vi "Execute.vi"(8 "error in (no error)":errorcluster, 9 "Workspace":T1, 10 "Control In":T2={"I-O.lvclass"=refnum, "Gantry"=refnum, "Dispenser"="COM1"}, 11 "Secure Syringe in":refnum<class "SecureRelease Syringe.lvclass">) -> (0 "error out":errorcluster, 2 "Control Out":T2={"I-O.lvclass"=refnum, "Gantry"=refnum, "Dispenser"="COM1"}, 3 "Secure Syringe out":refnum<class "SecureRelease Syringe.lvclass">)   [LabVIEW 2020, in "SecureRelease Syringe.lvclass"]
uses:
  SecureRelease Syringe.lvclass
  Controller/Controllers.ctl
  Controller/I-O/I-O.lvclass
  C:/Program Files (x86)/Aerotech/A3200/LabVIEW/2010/Bin/Aerotech.A3200.dll
  Program Files (x86)/Aerotech/A3200/LabVIEW/2010/Bin/Aerotech.A3200.dll
  Workspace/Workspace.ctl
  SecureRelease Syringe.lvclass/SecureRelease Syringe.ctl
  Controller/Motion/Motion.lvclass
  Dispense/Dispense.lvclass
  Controller/Motion/A3200/A3200.lvclass
  Controller/Dispenser/Dispenser.lvclass
  Controller/Controller.lvclass
  Workspace/Fixture.lvclass
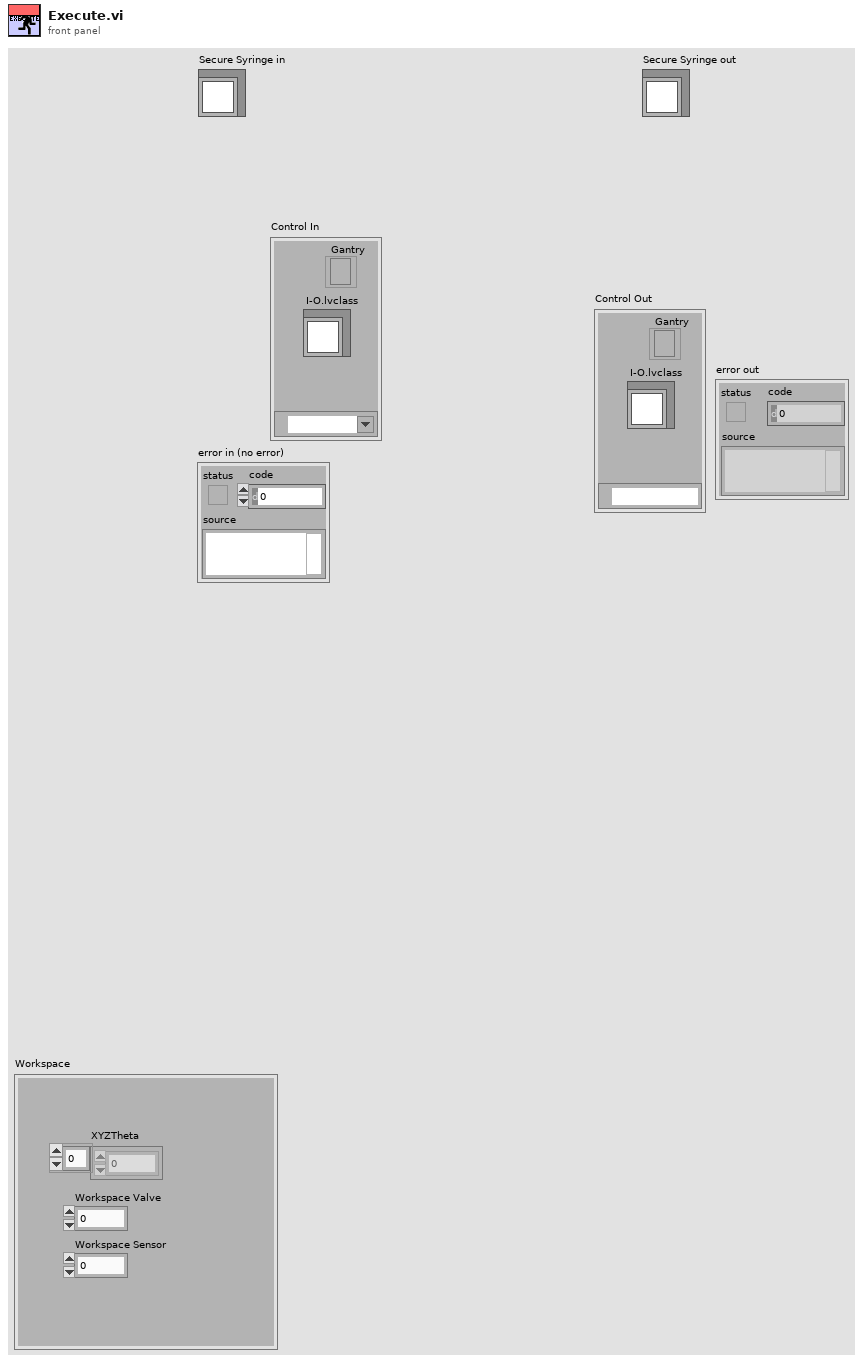
[diagram p1: front panel]
types:
  T1 = typedef "Fixture.lvclass/Workspace.ctl" = cluster{"XYZTheta":dbl[], "Workspace Valve":i32, "Workspace Sensor":i32}
  T2 = typedef "Controller.lvclass/Controllers.ctl" = cluster{"I-O.lvclass":refnum<class "I-O.lvclass">, "Gantry":refnum<k24>, "Dispenser":refnum<visa-resource-name>}
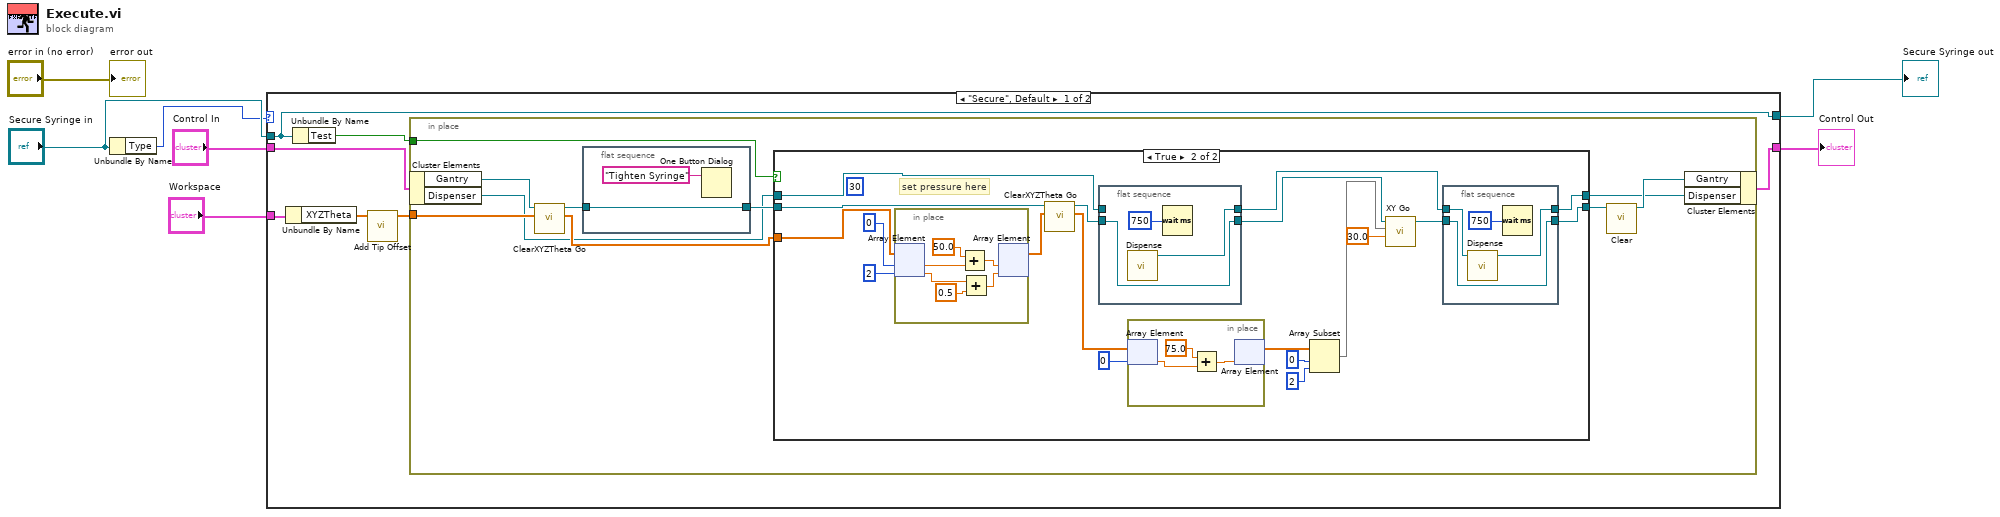
[diagram p0: block diagram]
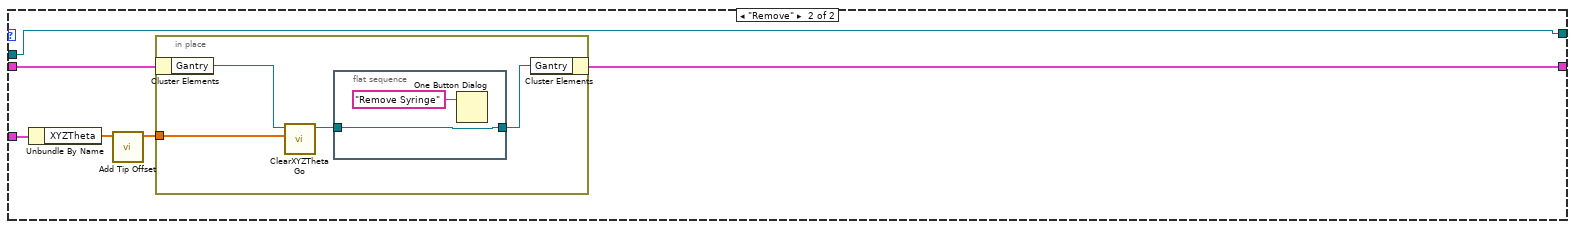
[diagram p3: hidden frame]
diagram:
  n1 = Unbundle By Name("Secure Syringe in") -> ("Type"=w1:enum16{"Secure", "Remove"})
  n2 = case shown="\"Secure\", Default" w1 {
    tunnel: "Workspace" -> [w14 w66]
    tunnel: "Secure Syringe in" -> [w10 w67]
    tunnel: [w10 w67] -> w5
    tunnel: "Control In" -> [w13 w68]
    tunnel: [w12 w69] -> w3
    frame "Secure", Default {
      n3 = Unbundle By Name(w14) -> ("XYZTheta"=w9:dbl[])
      n4 = Unbundle By Name(w10) -> ("Test"=w11:bool)
      n5 = call "Add Tip Offset.vi"("XYZTheta"=w9) -> ("XYZTheta"=w8:dbl[])  [unwired: 10 in]
      n6 = in-place {
        in-place-border: w8 -> [w23]
        in-place-border: w11 -> [w17]
        n7 = in-place-cluster #1(w13) -> ("Gantry"=w24:refnum<k24>, "Dispenser"=w16:refnum<visa-resource-name>)
        n8 = call "ClearXYZTheta Go.vi"("XYZTheta In"=w23, "Gantry In"=w24) -> ("XYZTheta Out"=w18:dbl[], "Gantry Out"=w22:refnum<k24>)  [unwired: 7 in, 1 out]
        n9 = flat-sequence {
          tunnel: [w62] -> w20
          tunnel: w22 -> [w62]
          frame #0 {
            n10 = One Button Dialog(message="Tighten Syringe") -> ()  [unwired: 1 in, 1 out]
          }
        }
        n11 = case shown="True" w17 {
          tunnel: w20 -> [w26 w45]
          tunnel: [w26 w37] -> w19
          tunnel: w18 -> [_ w44]
          tunnel: w16 -> [w25 w27]
          tunnel: [w25 w35] -> w15
          frame False {
          }
          frame True {
            (unwired) i16 30 ("Pressure")
            # "set pressure here"
            n12 = in-place {
              n13 = in-place-array #2(w44, 0, 2) -> (w61:dbl, w59:dbl)
              n14 = Add(x=50.0, y=w61) -> (x+y=w56:dbl)
              n15 = Add(x=w59, y=0.5) -> (x+y=w57:dbl)
              n16 = in-place-array #2(w56, w57) -> (w41:dbl[])  [unwired: 2 out]
            }
            n17 = call "ClearXYZTheta Go.vi"("XYZTheta In"=w41, "Gantry In"=w45) -> ("XYZTheta Out"=w40:dbl[], "Gantry Out"=w38:refnum<k24>)  [unwired: 7 in, 1 out]
            n18 = flat-sequence {
              tunnel: [w52] -> w29
              tunnel: w38 -> [w52]
              tunnel: w27 -> [_]
              tunnel: [w50] -> w36
              frame #0 {
                n19 = call "Dispense.vi"() -> ("Dispenser Out"=w50:refnum<visa-resource-name>)  [unwired: 10 in, 1 out]
                n20 = Wait (ms)(milliseconds to wait=u32 750) -> ()  [unwired: 1 out]
              }
            }
            n21 = in-place {
              n22 = in-place-array #3(w40, 0) -> (w55:dbl)
              n23 = Add(x=75.0, y=w55) -> (x+y=w53:dbl)
              n24 = in-place-array #3(w53) -> (w34:dbl[])  [unwired: 1 out]
            }
            n25 = Array Subset(array=w34, index=0, length=2) -> (w31:dbl[])
            n26 = call "XY Go.vi"("Speed"=30.0, "XY"=w31, "Gantry In"=w29) -> ("Gantry Out"=w28:refnum<k24>)  [unwired: 7 in, 1 out]
            n27 = flat-sequence {
              tunnel: [w49] -> w37
              tunnel: w28 -> [w49]
              tunnel: w36 -> [w46]
              tunnel: [w47] -> w35
              frame #0 {
                n28 = call "Dispense.vi"("Dispenser In"=w46) -> ("Dispenser Out"=w47:refnum<visa-resource-name>)  [unwired: 9 in, 1 out]
                n29 = Wait (ms)(milliseconds to wait=u32 750) -> ()  [unwired: 1 out]
              }
            }
          }
        }
        n30 = call "Clear.vi"("Gantry In"=w19) -> ("Gantry Out"=w21:refnum<k24>)  [unwired: 9 in, 1 out]
        n31 = in-place-cluster #1("Gantry"=w21, "Dispenser"=w15) -> (w12:T2)
      }
    }
    frame "Remove" {
      n32 = Unbundle By Name(w66) -> ("XYZTheta"=w65:dbl[])
      n33 = call "Add Tip Offset.vi"("XYZTheta"=w65) -> ("XYZTheta"=w64:dbl[])  [unwired: 10 in]
      n34 = in-place {
        in-place-border: w64 -> [w70]
        n35 = in-place-cluster #4(w68) -> ("Gantry"=w73:refnum<k24>)
        n36 = call "ClearXYZTheta Go.vi"("XYZTheta In"=w70, "Gantry In"=w73) -> ("Gantry Out"=w72:refnum<k24>)  [unwired: 7 in, 2 out]
        n37 = flat-sequence {
          tunnel: w72 -> [w75]
          tunnel: [w75] -> w71
          frame #0 {
            n38 = One Button Dialog(message="Remove Syringe") -> ()  [unwired: 1 in, 1 out]
          }
        }
        n39 = in-place-cluster #4("Gantry"=w71) -> (w69:T2)
      }
    }
  }
  "Secure Syringe out" <- w5
  "Control Out" <- w3
  "error out" <- "error in (no error)"
